vi "Read Stream and Create Channels.vi"(8 "error in (no error)":errorcluster, 10 "StreamReader Parameters in":T1, 11 "Plugin in":refnum<class "StreamReader.lvclass">) -> (0 "error out":errorcluster, 1 "Array":waveform(dbl)[](array[waveform]), 2 "StreamReader Parameters out":T1, 3 "Plugin out":refnum<class "StreamReader.lvclass">)   [LabVIEW 2024, in "StreamReader.lvlib" / "StreamReader.lvclass"]
uses:
  StreamReader.lvclass
  StreamReader Parameters.ctl
  <vilib>/FlexLogger/SDK/PluginSDK.lvlibp/PEFClasses/SDK/Producer Channel/Producer Channel.lvclass
  C:/Program Files/National Instruments/LabVIEW 2024/vi.lib/FlexLogger/SDK/PluginSDK.lvlibp/PEFClasses/SDK/Channel/Channel.lvclass
  <vilib>/FlexLogger/SDK/PluginSDK.lvlibp/PEFClasses/SDK/Producer Channel/Create Producer Channel.vi
  StreamReader.lvclass/StreamReader.ctl
  <vilib>/FlexLogger/SDK/PluginSDK.lvlibp
  <vilib>/FlexLogger/SDK/PluginSDK.lvlibp/PEFClasses/SDK/Plugin/Plugin.lvclass
  <resource>/objmgr/ni.dex.rc
  C:/Program Files/National Instruments/LabVIEW 2024/vi.lib/FlexLogger/SDK/PluginSDK.lvlibp/PEFClasses/SDK/Plugin/Plugin.lvclass
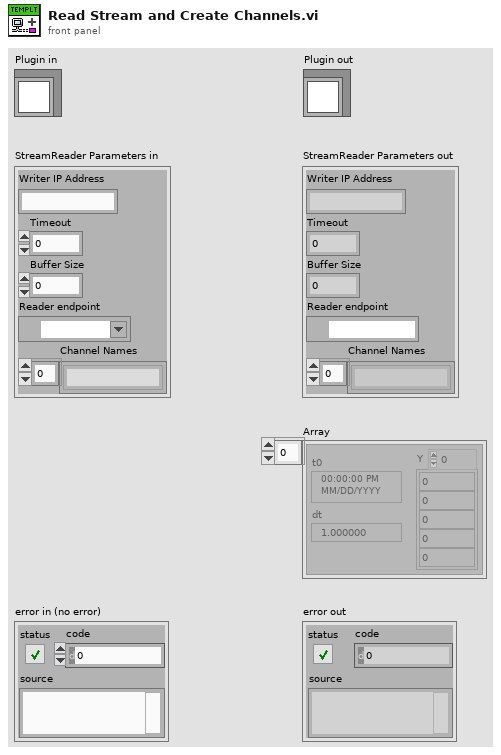
[diagram p1: front panel]
types:
  T1 = typedef "StreamReader.lvlib/StreamReader.lvclass/StreamReader Parameters.ctl" = cluster{"Writer IP Address":string, "Timeout":i32, "Buffer Size":i32, "Reader endpoint":refnum<k21>, "Channel Names":string[]}
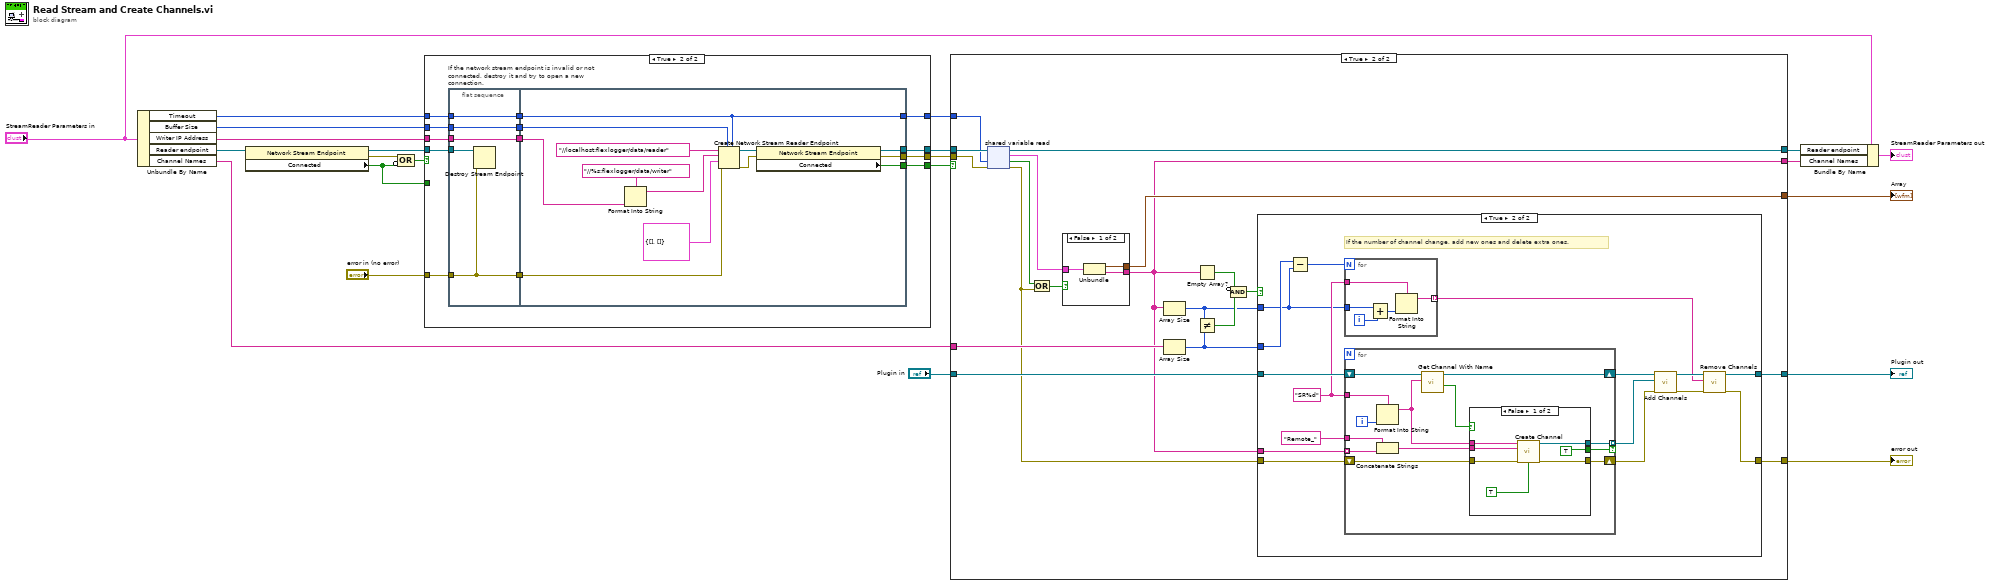
[diagram p0: block diagram]
diagram:
  n1 = Unbundle By Name("StreamReader Parameters in") -> ("Timeout"=w16:i32, "Buffer Size"=w17:i32, "Writer IP Address"=w18:string, "Reader endpoint"=w15:refnum<k21>, "Channel Names"=w7:string[])
  n2 = property class="Network Stream Endpoint"(reference=w15) -> (reference out=w12:refnum<k21>, error out=w14:errorcluster, "Connected"=w11:bool)  [unwired: 1 in]
  n3 = Compound Arithmetic op=OR(w14, invert w11) -> (w13:bool)
  n4 = case shown="True" w13 {
    tunnel: [w24 w39] -> w22
    tunnel: [w26 w38] -> w21
    tunnel: [w25 w37] -> w20
    tunnel: "error in (no error)" -> [w24 w36]
    tunnel: w18 -> [_ w35]
    tunnel: w17 -> [_ w34]
    tunnel: w16 -> [w23 w33]
    tunnel: w12 -> [w25 w28]
    tunnel: w11 -> [w26 _]
    tunnel: [w23 w27] -> w10
    frame False {
    }
    frame True {
      n5 = flat-sequence "If the network stream endpoint is invalid or not connected, destroy it and try to open a new connection." {
        tunnel: w33 -> [w42]
        tunnel: w34 -> [w43]
        tunnel: w35 -> [w44]
        tunnel: w36 -> [w40]
        tunnel: [w40] -> w32
        tunnel: [w44] -> w31
        tunnel: [w43] -> w30
        tunnel: [w42] -> w29
        tunnel: w28 -> [w41]
        tunnel: [w57] -> w39
        tunnel: [w56] -> w38
        tunnel: [w49] -> w37
        tunnel: w32 -> [w48]
        tunnel: w31 -> [w47]
        tunnel: w30 -> [w46]
        tunnel: w29 -> [w45]
        tunnel: [w45] -> w27
        frame #0 {
          n6 = Destroy Stream Endpoint(8:w40, 11:w41) -> ()  [unwired: 1 out]
        }
        frame #1 {
          n7 = Format Into String(format string="//%s:flexlogger/data/writer" ("reader url"), w47) -> (resulting string=w51:string)  [unwired: 2 in, 1 out]
          n8 = Create Network Stream Reader Endpoint(5:w45, 7:w46, 8:w48, 9:cluster{waveform(dbl)[], string[]} {[], []}, 10:w51, 11:"//localhost:flexlogger/data/reader" ("writer name")) -> (0:w52:errorcluster, 3:w55:refnum<k21>)  [unwired: 1 in]
          n9 = property class="Network Stream Endpoint"(reference=w55, error in=w52) -> (reference out=w49:refnum<k21>, error out=w57:errorcluster, "Connected"=w56:bool)
        }
      }
    }
  }
  n10 = case shown="True" w21 {
    tunnel: w20 -> [w60 w78]
    tunnel: w22 -> [w61 w77]
    tunnel: w10 -> [_ w75]
    tunnel: [w61 w67] -> w5
    tunnel: [w60 w74] -> w3
    tunnel: "Plugin in" -> [w59 w69]
    tunnel: [w59 w68] -> w8
    tunnel: w7 -> [w58 w66]
    tunnel: [_ w73] -> w6
    tunnel: [w58 w65] -> w2
    frame False {
    }
    frame True {
      n11 = shared-variable-read(w78, w77, w75) -> (w74:refnum<k21>, w62:errorcluster, w79:bool, w80:cluster{waveform(dbl)[], string[]})
      n12 = Or(x=w79, y=w62) -> (x .or. y?=w76:bool)
      n13 = case shown="False" w76 {
        tunnel: w80 -> [w127 _]
        tunnel: [w126 _] -> w65
        tunnel: [w125 _] -> w73
        frame False {
          n14 = Unbundle(w127) -> (w125:waveform(dbl)[], w126:string[])
        }
        frame True {
        }
      }
      n15 = Array Size(array=w65) -> (size(s)=w63:i32)
      n16 = Array Size(array=w66) -> (size(s)=w64:i32)
      n17 = Empty Array?(array=w65) -> (empty?=w72:bool)
      n18 = Not Equal?(x=w63, y=w64) -> (x != y?=w71:bool)
      n19 = Compound Arithmetic op=AND(invert w72, w71) -> (w70:bool)
      n20 = case shown="True" w70 {
        tunnel: w62 -> [w82 w96]
        tunnel: [w82 w91] -> w67
        tunnel: w69 -> [w81 w90]
        tunnel: w65 -> [_ w95]
        tunnel: [w81 w89] -> w68
        tunnel: w64 -> [_ w87]
        tunnel: w63 -> [_ w84]
        frame False {
        }
        frame True {
          w85 = "SR%d" ("format string")
          # "If the number of channel change, add new ones and delete extra ones."
          n21 = Subtract(x=w87, y=w84) -> (x-y=w86:i32)
          n22 = for {
            N: w86 -> [_]
            tunnel: w85 -> [w103]
            tunnel: w84 -> [w102]
            tunnel: [w99] -> w83 mode=indexing
            i -> [w101]
            n23 = Add(x=w102, y=w101) -> (x+y=w100:i32)
            n24 = Format Into String(format string=w103, w100) -> (resulting string=w99:string)  [unwired: 2 in, 1 out]
          }
          n25 = for {
            tunnel: w95 -> [w113] mode=indexing
            shift-right: [w115] -> w97
            shift-left: w96 -> [w116]
            tunnel: [w114] -> w98 mode=indexing if=w110
            shift-right: [w107] -> w94
            shift-left: w90 -> [w108]
            tunnel: "Remote_" ("string") -> [w105]
            tunnel: w85 -> [w104]
            i -> [w109]
            n26 = Format Into String(format string=w104, w109) -> (resulting string=w106:string)  [unwired: 2 in, 1 out]
            n27 = Concatenate Strings(w105, w113) -> (w112:string)
            n28 = call <vilib>:"Get Channel With Name.vi"("Name"=w106, "Plugin in"=w108) -> ("Found?"=w111:bool, "Plugin out"=w107:refnum<class "StreamReader.lvclass">)  [unwired: 7 in, 1 out]
            n29 = case shown="False" w111 {
              tunnel: w116 -> [w122 w124]
              tunnel: [w121 w124] -> w115
              tunnel: [w120 _] -> w114
              tunnel: w112 -> [w119 _]
              tunnel: w106 -> [w118 _]
              tunnel: [TRUE _] -> w110
              frame False {
                n30 = call-poly <vilib>:"Create Channel.vi"("Unique Channel Identifier"=w118, "Default Channel Name"=w119, "error in (no error)"=w122, "Can Disable?"=TRUE) -> ("Producer Channel"=w120:refnum<class "Producer Channel.lvclass">, "error out"=w121:errorcluster)  [unwired: 10 in]
              }
              frame True {
              }
            }
          }
          n31 = call <vilib>:"Add Channels.vi"("error in (no error)"=w97, "Channels"=w98, "Plugin in"=w94) -> ("error out"=w93:errorcluster, "Plugin out"=w92:refnum<class "StreamReader.lvclass">)  [unwired: 7 in]
          n32 = call-dynamic "Remove Channels.vi"("error in (no error)"=w93, "Unique Channel Identifiers to Delete"=w83, "Plugin in"=w92) -> ("error out"=w91:errorcluster, "Plugin out"=w89:refnum<class "StreamReader.lvclass">)  [unwired: 7 in]
        }
      }
    }
  }
  "error out" <- w5
  "Plugin out" <- w8
  "Array" <- w6
  n33 = Bundle By Name(cluster="StreamReader Parameters in", "Reader endpoint"=w3, "Channel Names"=w2) -> (→"StreamReader Parameters out":T1)
